vi "Close VI.vi"(10 "Log File Cluster":T1) -> (2 "State Ring":u16(ring) items=["Init VI", "Init Event Handlers", "Booting sequence", "Operational", "Emergency shutting down", "Shuting down", "Closing VI"])   [LabVIEW 2016]
uses:
  Log File Cluster.ctl
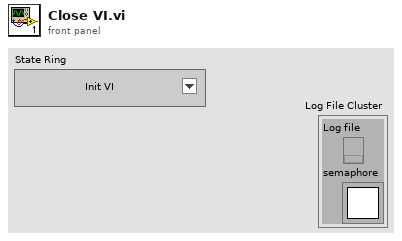
[diagram p1: front panel]
types:
  T1 = typedef "Log File Cluster.ctl" = cluster{"Log file":refnum<k34>, "semaphore":T2}
  T2 = typedef "Semaphore RefNum" = refnum<k1>
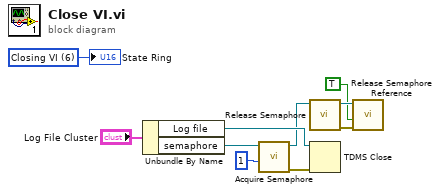
[diagram p0: block diagram]
diagram:
  w2 = u16 6 items=["Init VI", "Init Event Handlers", "Booting sequence", "Operational", "Emergency shutting down", "Shuting down", "Closing VI"] ("State Ring")
  n1 = Unbundle By Name("Log File Cluster") -> ("Log file"=w10:refnum<k34>, "semaphore"=w9:T2)
  n2 = call <vilib>:"Acquire Semaphore.vi"("ms timeout (-1)"=1, "semaphore"=w9) -> ("error out"=w8:errorcluster, "semaphore out"=w6:T2)  [unwired: 3 in, 1 out]
  n3 = call <vilib>:"Release Semaphore.vi"("semaphore"=w6) -> ("error out"=w4:errorcluster, "semaphore out"=w5:T2)  [unwired: 5 in]
  n4 = TDMS Close(8:w8, 11:w10) -> ()  [unwired: 2 out]
  n5 = call <vilib>:"Release Semaphore Reference.vi"("error in (no error)"=w4, "force destroy? (F)"=TRUE, "semaphore"=w5) -> ()  [unwired: 7 in, 2 out]
  "State Ring" <- w2
